vi "Station1_Data_Log.vi"(8 "error in (no error)":errorcluster, 10 "Para In":T1, 11 "Cluster":T3) -> (0 "error out":errorcluster)   [LabVIEW 2017]
uses:
  <vilib>/addons/database/Connection.llb/Conn ObjectReference.ctl
  <vilib>/addons/database/NI_Database_API.lvlib
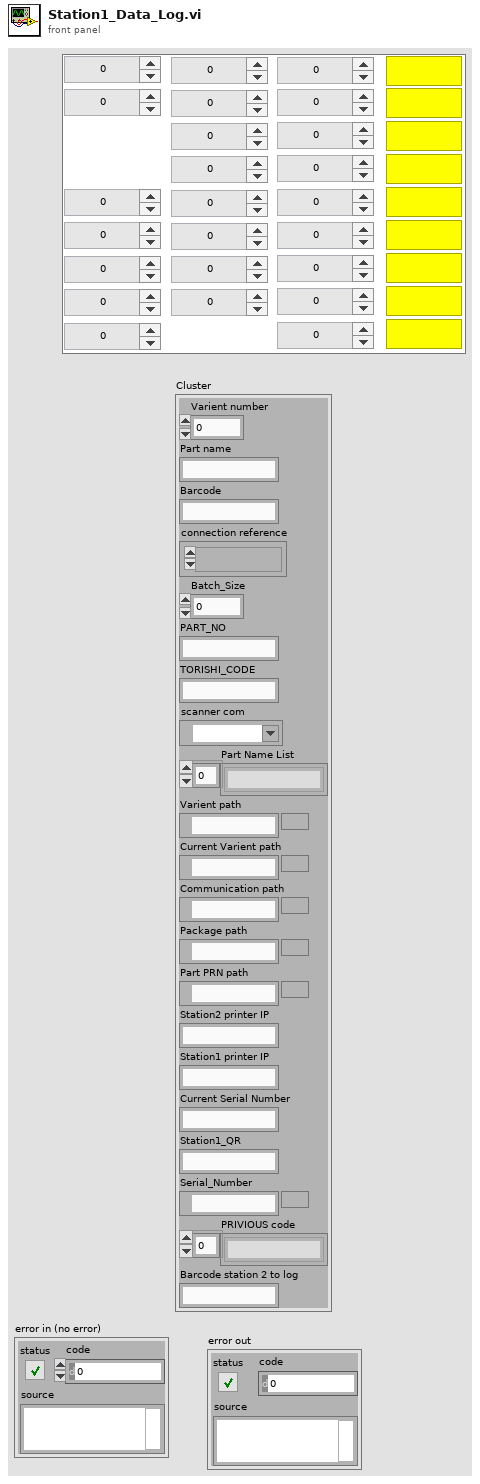
[diagram p1: front panel]
types:
  T1 = cluster{"1.1":dbl, "1.2":dbl, "1.3":dbl, "2.1":dbl, "2.2":dbl, "2.3":dbl, "3.2":dbl, "3.3":dbl, "4.2":dbl, "4.3":dbl, "5.1":dbl, "5.2":dbl, "5.3":dbl, "6.1":dbl, "6.2":dbl, "6.3":dbl, "7.1":dbl, "7.2":dbl, "7.3":dbl, "8.1":dbl, "8.2":dbl, "8.3":dbl, "9.1":dbl, "9.3":dbl, "1.4 CYCLE START":bool, "2.4 CYCLE START":bool, "3.4 CYCLE START":bool, "4.4 CYCLE START":bool, "5.4 CYCLE START":bool, "6.4 CYCLE START":bool, "7.4 CYCLE START":bool, "8.4 CYCLE START":bool, "9.4 CYCLE START":bool}
  T2 = typedef "NI_Database_API.lvlib/Conn ObjectReference.ctl" = refnum<k1>
  T3 = cluster{"Varient number":u16, "Part name":string, "Barcode":string, "connection reference":T2, "Batch_Size":u16, "PART_NO":string, "TORISHI_CODE":string, "scanner com":refnum<visa-resource-name>, "Part Name List":string[], "Varient path":path, "Current Varient path":path, "Communication path":path, "Package path":path, "Part PRN path":path, "Station2 printer IP":string, "Station1 printer IP":string, "Current Serial Number":string, "Station1_QR":string, "Serial_Number":path, "PRIVIOUS code":string[], "Barcode station 2 to log":string}
  T4 = cluster{string, string, string, "Part name":string, "PART_NO":string, "TORISHI_CODE":string, string, string, "station1 rst":string, string, "Current Serial Number":string, "Station1_QR":string, "9.3":string, "9.3":string, "9.3":string, string, "9.3":string, "9.3":string, "9.3":string, string, "9.3":string, "9.3":string, string, "9.3":string, "9.3":string, string, "9.3":string, "9.3":string, "9.3":string, string, "9.3":string, "9.3":string, "9.3":string, string, "9.3":string, "9.3":string, "9.3":string, string, "9.3":string, "9.3":string, "9.3":string, string, "9.3":string, "9.3":string, string}
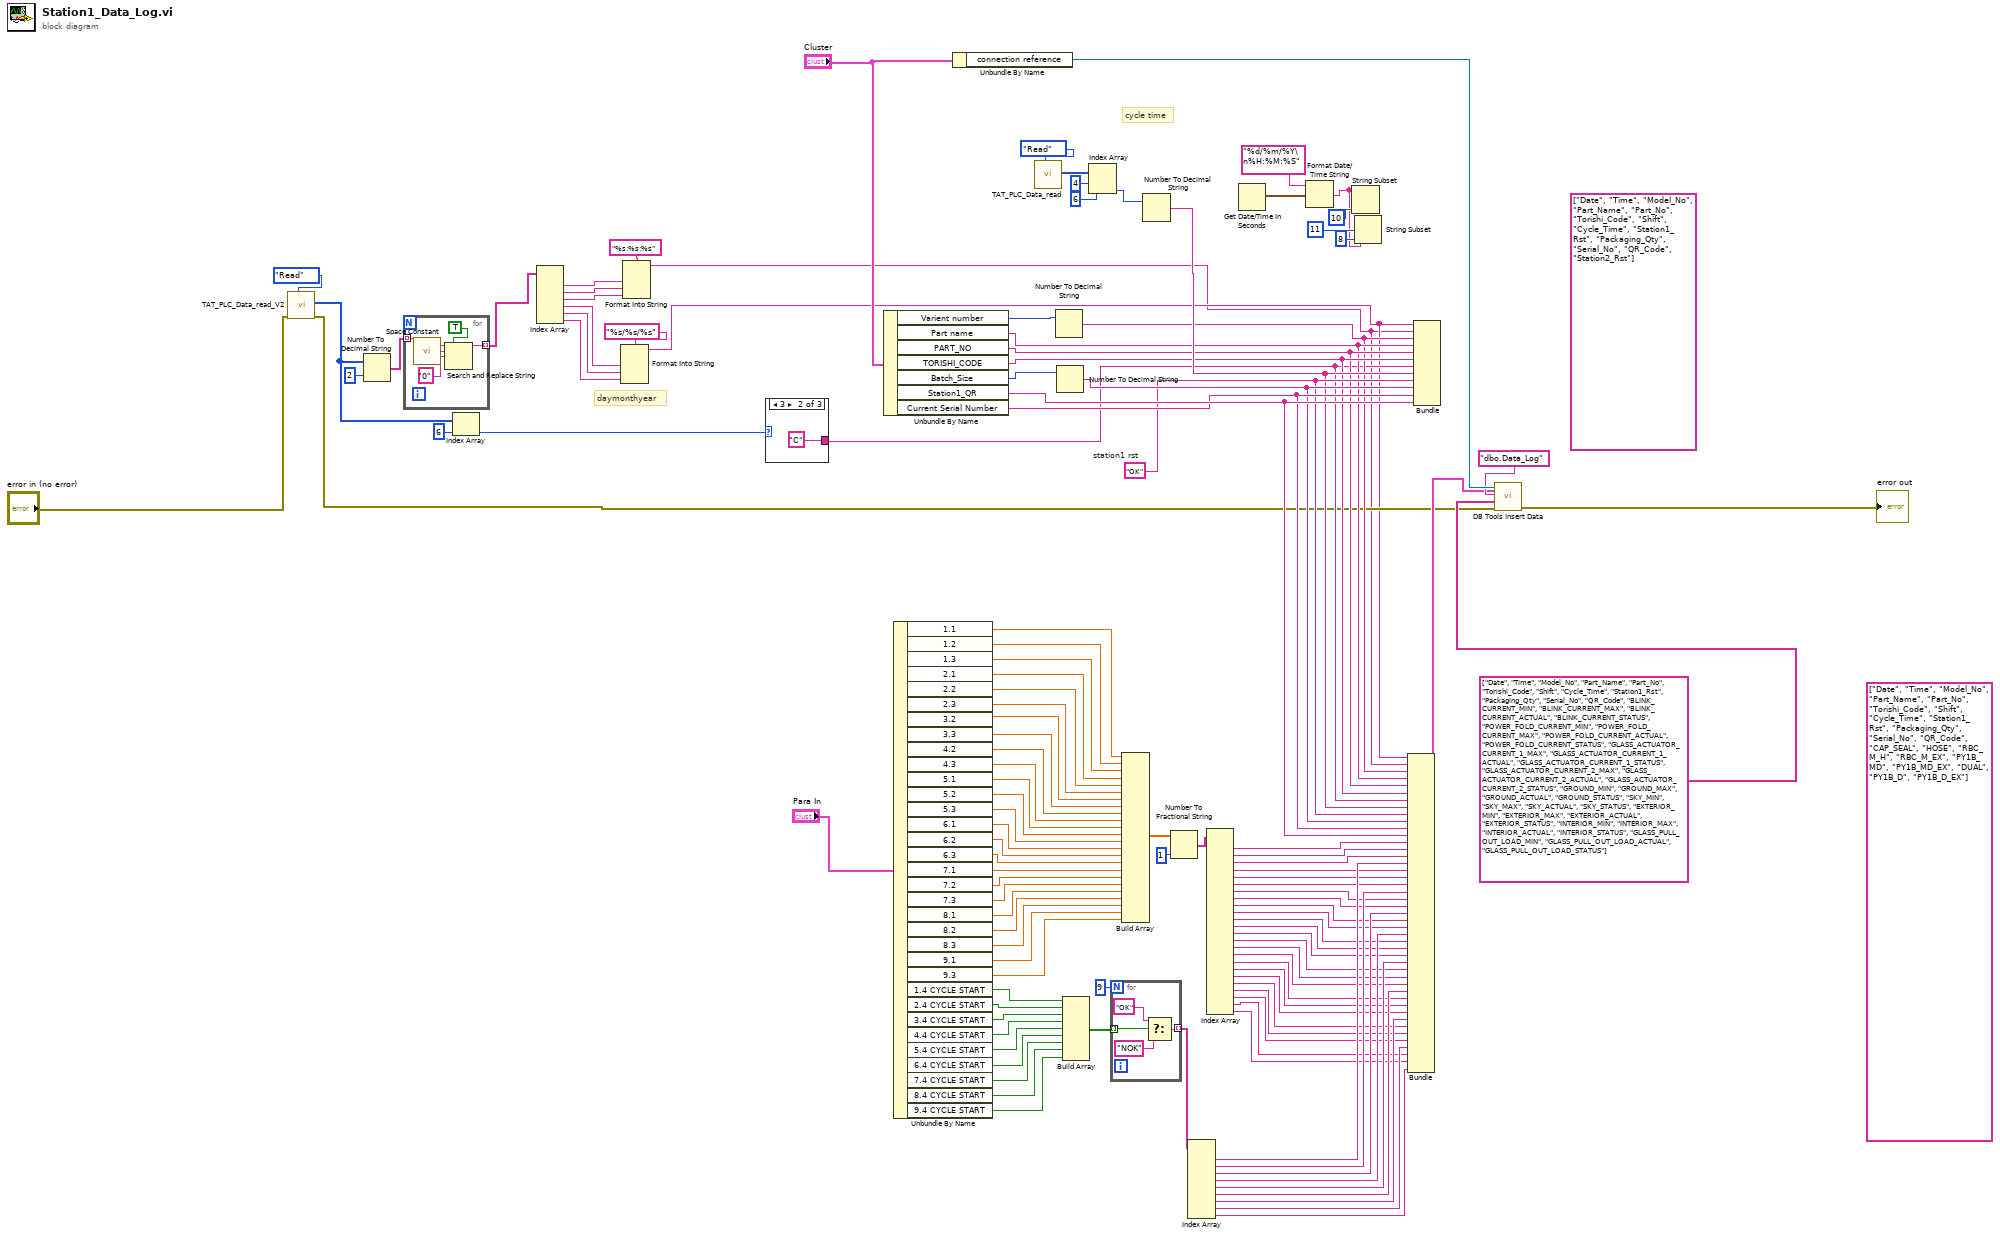
[diagram p0: block diagram]
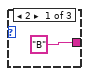
[diagram p2: hidden frame]
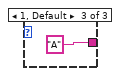
[diagram p3: hidden frame]
diagram:
  w27 = "OK"  # station1 rst
  (unwired) string[] ["Date", "Time", "Model_No", "Part_Name", "Part_No", "Torishi_Code", "Shift", "Cycle_Time", "Station1_Rst", "Packaging_Qty", "Serial_No", "QR_Code", "Station2_Rst"] ("columns 2")
  (unwired) string[] ["Date", "Time", "Model_No", "Part_Name", "Part_No", "Torishi_Code", "Shift", "Cycle_Time", "Station1_Rst", "Packaging_Qty", "Serial_No", "QR_Code", "CAP_SEAL", "HOSE", "RBC_M_H", "RBC_M_EX", "PY1B_MD", "PY1B_MD_EX", "DUAL", "PY1B_D", "PY1B_D_EX"] ("columns 2")
  # "daymonthyear"
  # "cycle time"
  n1 = call "TAT_PLC_Data_read_V2.vi"("Enum"=enum16{"Read", "Write"}."Read", "error in (no error)"="error in (no error)") -> ("error out"=w9:errorcluster, "Array 2"=w2:u16[])  [unwired: 8 in]
  n2 = Number To Decimal String(number=w2, width (-)=i16 2) -> (decimal integer string=w5:string[])
  n3 = for {
    tunnel: w5 -> [w123] mode=indexing
    tunnel: [w122] -> w4 mode=indexing
    n4 = call <vilib>:"Space Constant.vi"() -> ("String"=w124:string)
    n5 = Search and Replace String(replace all?=TRUE ("replace all? (F)"), input string=w123, search string=w124, replace string="0" ("replace string (\"\")")) -> (result string=w122:string)  [unwired: 4 in, 3 out]
  }
  n6 = Index Array(array=w2, index=6) -> (element=w1:u16)
  n7 = Index Array(array=w4) -> (element #1=w14:string, element #2=w13:string, element #3=w12:string, element #4=w18:string, element #5=w20:string, element #6=w19:string)  [unwired: 6 in]
  n8 = Format Into String(format string="%s/%s/%s" ("time format string (%c)"), w18, w20, w19) -> (resulting string=w8:string)  [unwired: 2 in, 1 out]
  n9 = Format Into String(format string="%s:%s:%s" ("time format string (%c)"), w14, w13, w12) -> (resulting string=w7:string)  [unwired: 2 in, 1 out]
  n10 = case shown="3" w1 {
    tunnel: ["B" "C" "A"] -> w11
    frame 2 {
    }
    frame 3 {
    }
    frame 1, Default {
    }
  }
  n11 = Unbundle By Name("Cluster") -> ("Varient number"=w120:u16, "Part name"=w23:string, "PART_NO"=w24:string, "TORISHI_CODE"=w25:string, "Batch_Size"=w121:u16, "Station1_QR"=w30:string, "Current Serial Number"=w29:string)
  n12 = Unbundle By Name("Para In") -> ("1.1"=w89:dbl, "1.2"=w88:dbl, "1.3"=w87:dbl, "2.1"=w86:dbl, "2.2"=w85:dbl, "2.3"=w84:dbl, "3.2"=w83:dbl, "3.3"=w82:dbl, "4.2"=w81:dbl, "4.3"=w80:dbl, "5.1"=w79:dbl, "5.2"=w78:dbl, "5.3"=w77:dbl, "6.1"=w76:dbl, "6.2"=w75:dbl, "6.3"=w74:dbl, "7.1"=w73:dbl, "7.2"=w72:dbl, "7.3"=w71:dbl, "8.1"=w70:dbl, "8.2"=w69:dbl, "8.3"=w68:dbl, "9.1"=w67:dbl, "9.3"=w66:dbl, "1.4 CYCLE START"=w100:bool, "2.4 CYCLE START"=w99:bool, "3.4 CYCLE START"=w98:bool, "4.4 CYCLE START"=w97:bool, "5.4 CYCLE START"=w96:bool, "6.4 CYCLE START"=w95:bool, "7.4 CYCLE START"=w94:bool, "8.4 CYCLE START"=w93:bool, "9.4 CYCLE START"=w92:bool)
  n13 = Unbundle By Name("Cluster") -> ("connection reference"=w113:T2)
  n14 = call "TAT_PLC_Data_read.vi"("Enum"=enum16{"Read", "Write"}."Read") -> ("Array 2"=w110:u16[])  [unwired: 9 in, 1 out]
  n15 = Number To Decimal String(number=w120) -> (decimal integer string=w22:string)  [unwired: 1 in]
  n16 = Number To Decimal String(number=w121) -> (decimal integer string=w28:string)  [unwired: 1 in]
  n17 = Build Array(w100, w99, w98, w97, w96, w95, w94, w93, w92) -> (w91:bool[])
  n18 = Index Array(array=w110, index #1=4 ("index"), index #2=6 ("index")) -> (element #2=w106:u16)  [unwired: 1 out]
  n19 = for {
    N: 9 ("index") -> [_]
    tunnel: [w131] -> w102 mode=indexing
    tunnel: w91 -> [w130] mode=indexing
    n20 = Select(t="OK", s=w130, f="NOK") -> (s? t:f=w131:string)
  }
  n21 = Build Array(w89, w88, w87, w86, w85, w84, w83, w82, w81, w80, w79, w78, w77, w76, w75, w74, w73, w72, w71, w70, w69, w68, w67, w66) -> (w65:dbl[])
  n22 = Number To Decimal String(number=w106) -> (decimal integer string=w26:string)  [unwired: 1 in]
  n23 = Number To Fractional String(number=w65, precision (6)=i16 1) -> (F-format string=w64:string[])  [unwired: 2 in]
  n24 = Index Array(array=w102) -> (element #1=w60:string, element #2=w56:string, element #3=w53:string, element #4=w50:string, element #5=w46:string, element #6=w42:string, element #7=w38:string, element #8=w34:string, element #9=w31:string)  [unwired: 9 in]
  n25 = Index Array(array=w64) -> (element #1=w63:string, element #2=w62:string, element #3=w61:string, element #4=w59:string, element #5=w58:string, element #6=w57:string, element #7=w55:string, element #8=w54:string, element #9=w52:string, element #10=w51:string, element #11=w49:string, element #12=w48:string, element #13=w47:string, element #14=w45:string, element #15=w44:string, element #16=w43:string, element #17=w41:string, element #18=w40:string, element #19=w39:string, element #20=w37:string, element #21=w36:string, element #22=w35:string, element #23=w33:string, element #24=w32:string)  [unwired: 24 in]
  n26 = Get Date/Time In Seconds() -> (seconds since 1Jan1904=w114:timestamp)
  n27 = Format Date/Time String(time format string (%c)="%d/%m/%Y\n%H:%M:%S", seconds (now)=w114) -> (date/time string=w116:string)  [unwired: 1 in]
  n28 = String Subset(string=w116, length (rest)=10 ("length (rest)")) -> ()  [unwired: 1 in, 1 out]
  n29 = String Subset(string=w116, offset (0)=11 ("length (rest)"), length (rest)=8 ("length (rest)")) -> ()  [unwired: 1 out]
  n30 = Bundle(w8, w7, w22, "Part name"=w23, "PART_NO"=w24, "TORISHI_CODE"=w25, w11, w26, "station1 rst"=w27, w28, "Current Serial Number"=w29, "Station1_QR"=w30, "9.3"=w63, "9.3"=w62, "9.3"=w61, w60, "9.3"=w59, "9.3"=w58, "9.3"=w57, w56, "9.3"=w55, "9.3"=w54, w53, "9.3"=w52, "9.3"=w51, w50, "9.3"=w49, "9.3"=w48, "9.3"=w47, w46, "9.3"=w45, "9.3"=w44, "9.3"=w43, w42, "9.3"=w41, "9.3"=w40, "9.3"=w39, w38, "9.3"=w37, "9.3"=w36, "9.3"=w35, w34, "9.3"=w33, "9.3"=w32, w31) -> (w21:T4)  [unwired: 1 in]
  n31 = Bundle(w8, w7, w22, "Part name"=w23, "PART_NO"=w24, "TORISHI_CODE"=w25, w11, w26, "station1 rst"=w27, w28, "Current Serial Number"=w29, "Station1_QR"=w30) -> ()  [unwired: 1 in, 1 out]
  n32 = call <vilib>:"DB Tools Insert Data.vi"("data"=w21, "error in (no error)"=w9, "columns"=string[] ["Date", "Time", "Model_No", "Part_Name", "Part_No", "Torishi_Code", "Shift", "Cycle_Time", "Station1_Rst", "Packaging_Qty", "Serial_No", "QR_Code", "BLINK_CURRENT_MIN", "BLINK_CURRENT_MAX", "BLINK_CURRENT_ACTUAL", "BLINK_CURRENT_STATUS", "POWER_FOLD_CURRENT_MIN", "POWER_FOLD_CURRENT_MAX", "POWER_FOLD_CURRENT_ACTUAL", "POWER_FOLD_CURRENT_STATUS", "GLASS_ACTUATOR_CURRENT_1_MAX", "GLASS_ACTUATOR_CURRENT_1_ACTUAL", "GLASS_ACTUATOR_CURRENT_1_STATUS", "GLASS_ACTUATOR_CURRENT_2_MAX", "GLASS_ACTUATOR_CURRENT_2_ACTUAL", "GLASS_ACTUATOR_CURRENT_2_STATUS", "GROUND_MIN", "GROUND_MAX", "GROUND_ACTUAL", "GROUND_STATUS", "SKY_MIN", "SKY_MAX", "SKY_ACTUAL", "SKY_STATUS", "EXTERIOR_MIN", "EXTERIOR_MAX", "EXTERIOR_ACTUAL", "EXTERIOR_STATUS", "INTERIOR_MIN", "INTERIOR_MAX", "INTERIOR_ACTUAL", "INTERIOR_STATUS", "GLASS_PULL_OUT_LOAD_MIN", "GLASS_PULL_OUT_LOAD_ACTUAL", "GLASS_PULL_OUT_LOAD_STATUS"], "table"="dbo.Data_Log", "connection reference"=w113) -> ("error out"=→"error out":errorcluster)  [unwired: 5 in, 1 out]
